vi "Validate ROI arrays.vi"(7 "[ROI vis]":refnum<vi>, 9 "Old Value":T1 caption="Old value" {"ROI number" min=1 format="ROI %.0f"}, 11 "New Value":T1 caption="New value" {"ROI number" min=1 format="ROI %.0f"}) -> (0 "error out":errorcluster, 3 "[ROI #] out":T1 caption="Selected POI" {"ROI number" min=1 format="ROI %.0f"})   [LabVIEW 2013]
uses:
  Typedefs/ROI selector array-ROI vis.ctl
  xcontrol/Interface VIs/Interface typedefs/Interface-ROI selection cluster.ctl
  Typedefs/ROI ID Enum.ctl
  Typedefs/Get-Set-Clear Control.ctl
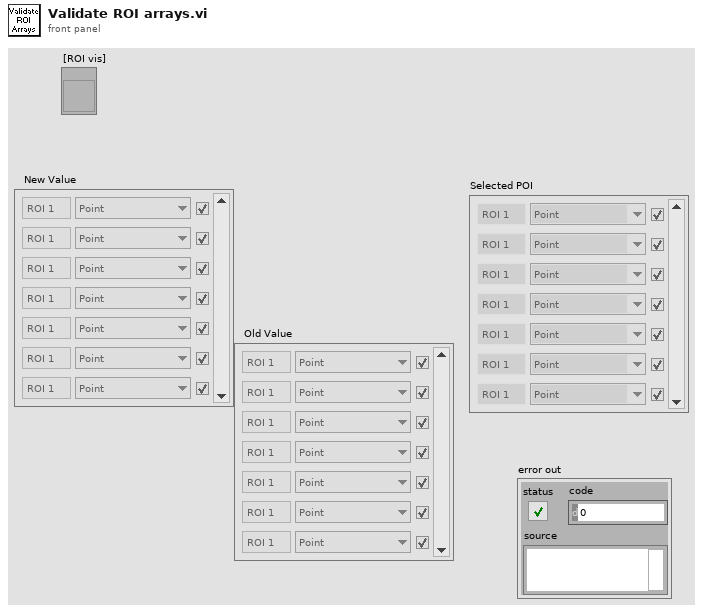
[diagram p1: front panel]
types:
  T1 = typedef "ROI selector array-ROI vis.ctl" = T2[]
  T2 = typedef "Interface-ROI selection cluster.ctl" = cluster{"ROI number":i32, "ROI ID":T3, "Visibility":bool}
  T3 = typedef "ROI ID Enum.ctl" = enum16{"Point", "MiniScan", "Comp. MiniScan", "Rectangle", "Comp. volume", "Arb. plane point"}
  T4 = cluster{"ROI number":i32, "ROI ID":T3, "Visibility":bool}
  T5 = cluster{"ROI number":i32, "ROI ID":T3, "Visibility":bool}[]
  T6 = cluster{"ROI index changed":bool, "ROI ID":bool, "Visibility changed":bool}
  T7 = typedef "Get-Set-Clear Control.ctl" = enum16{"Get", "Set", "Clear"}
  T8 = cluster{"ROI number":bool, "ROI ID":bool, "Visibility":bool}[]
  T9 = typedef "ROI indexes by type.ctl" = cluster{"Indexes of POI":i32[], "Indexes of Miniscans":i32[], "Indexes of? (Provisional)":i32[]}
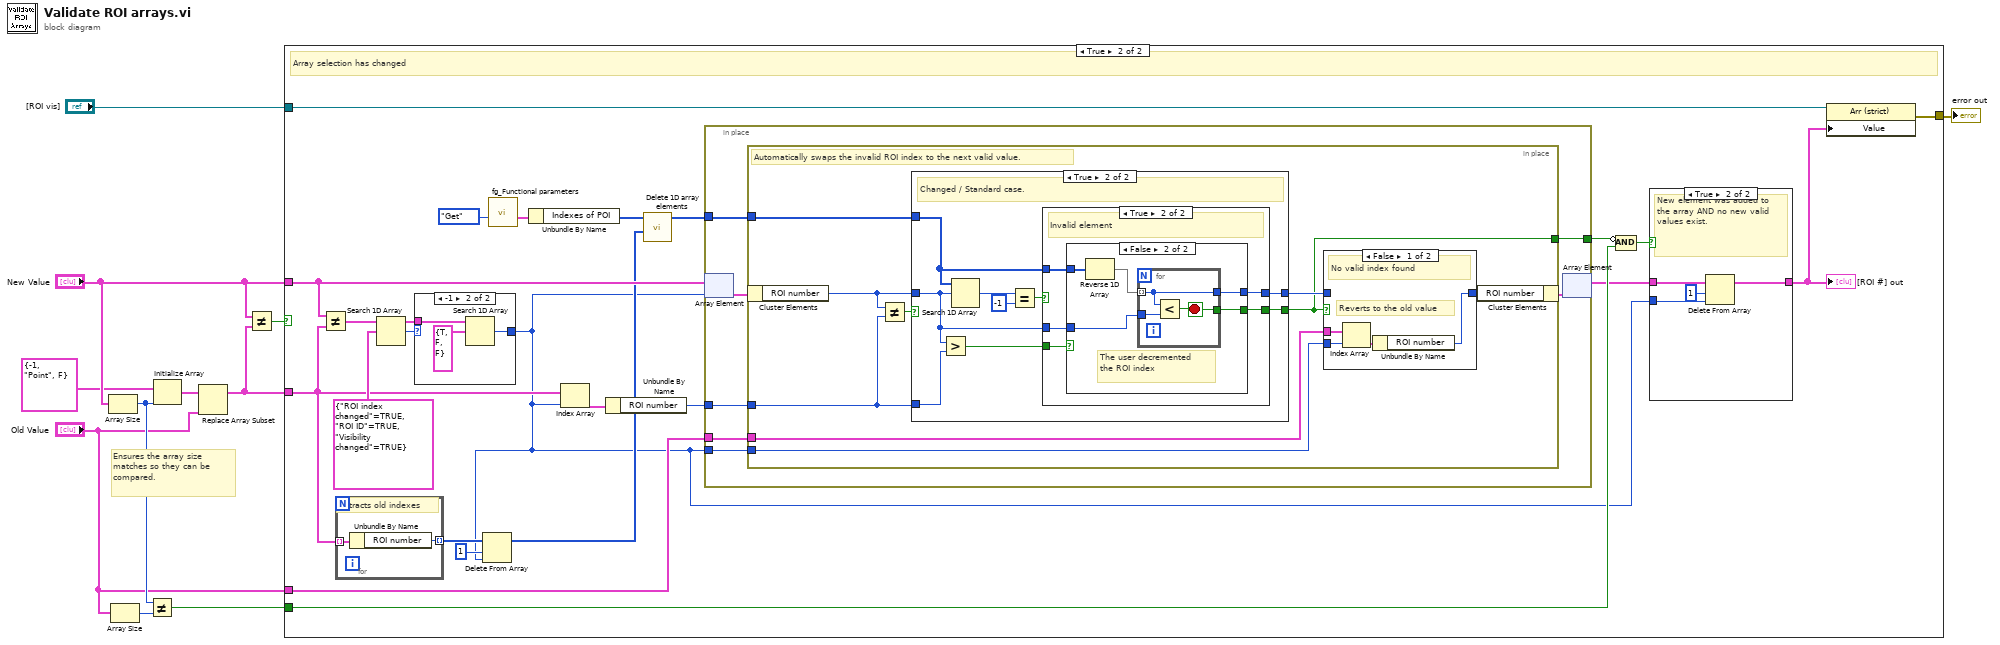
[diagram p0: block diagram]
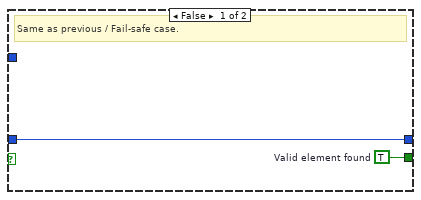
[diagram p5: hidden frame]
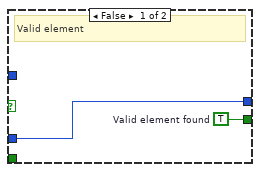
[diagram p6: hidden frame]
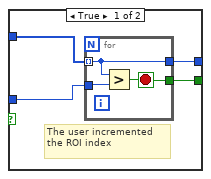
[diagram p7: hidden frame]
diagram:
  # "Ensures the array size matches so they can be compared."
  n1 = Array Size(array="New Value") -> (size(s)=w7:i32)
  n2 = Array Size(array="Old Value") -> (size(s)=w6:i32)
  n3 = Not Equal?(x=w7, y=w6) -> (x != y?=w5:bool)
  n4 = Initialize Array(T4 {"ROI number"=-1, "ROI ID"=enum."Point", "Visibility"=FALSE} ("System Cluster"), w7) -> (w10:T5)
  n5 = Replace Array Subset(array=w10, new element="Old Value") -> (w9:T5)  [unwired: 1 in]
  n6 = Not Equal?(x="New Value", y=w9) -> (x != y?=w11:bool)
  n7 = case shown="True" w11 {
    tunnel: "[ROI vis]" -> [_ w32]
    tunnel: "New Value" -> [_ w26]
    tunnel: w9 -> [_ w25]
    tunnel: w5 -> [_ w19]
    tunnel: "Old Value" -> [_ w14]
    tunnel: [_ w13] -> w3
    frame False {
      # "No change"
    }
    frame True {
      # "Array selection has changed"
      n8 = Not Equal?(x=w26, y=w25) -> (x != y?=w29:T8)
      n9 = for {
        tunnel: w25 -> [w41] mode=indexing
        tunnel: [w40] -> w24 mode=indexing
        # "Extracts old indexes"
        n10 = Unbundle By Name(w41) -> ("ROI number"=w40:i32)
      }
      n11 = Search 1D Array(1D array=w29, element=T6 {"ROI index changed"=TRUE, "ROI ID"=TRUE, "Visibility changed"=TRUE} ("POI sel & vis")) -> (index of element=w30:i32)  [unwired: 1 in]
      n12 = case shown="-1" w30 {
        selector: w30 -> [w96 _]
        tunnel: w29 -> [_ w99]
        tunnel: [w96 w98] -> w12
        frame Default {
        }
        frame -1 {
          n13 = Search 1D Array(1D array=w99, element=T6 {"ROI index changed"=TRUE, "ROI ID"=FALSE, "Visibility changed"=FALSE} ("POI sel & vis")) -> (index of element=w98:i32)  [unwired: 1 in]
        }
      }
      n14 = Delete From Array "Delete From Array"(array=w24, length=1, index=w12) -> (array with subset deleted=w22:i32[])  [unwired: 1 out]
      n15 = call "fg_Functional parameters.vi"("Function"=Get-Set-Clear_Control."Get") -> ("ROI indexes by type"=w33:T9)  [unwired: 7 in, 3 out]
      n16 = Unbundle By Name(w33) -> ("Indexes of POI"=w20:i32[])
      n17 = Index Array(array=w25, index=w12) -> (element=w28:T4)
      n18 = Unbundle By Name(w28) -> ("ROI number"=w27:i32)
      n19 = call "Delete 1D array elements.vi"("Elements to delete"=w22, "Input array"=w20) -> ("Array w elements deleted"=w21:i32[])  [unwired: 9 in]
      n20 = in-place {
        in-place-border: w21 -> [w48]
        in-place-border: w27 -> [w45]
        in-place-border: w14 -> [w44]
        in-place-border: w12 -> [w43]
        in-place-border: [w42] -> w18
        n21 = in-place-array #1(w26, w12) -> (w47:T2)
        n22 = in-place {
          in-place-border: w48 -> [w54]
          in-place-border: w45 -> [w55]
          in-place-border: w44 -> [w53]
          in-place-border: w43 -> [w52]
          in-place-border: [w49] -> w42
          # "Automatically swaps the invalid ROI index to the next valid value."
          n23 = in-place-cluster #2(w47) -> ("ROI number"=w57:i32)
          n24 = Not Equal?(x=w57, y=w55) -> (x != y?=w56:bool)
          n25 = case shown="True" w56 {
            tunnel: [w64 w70] -> w51
            tunnel: w54 -> [_ w69]
            tunnel: w57 -> [w64 w68]
            tunnel: w55 -> [_ w67]
            tunnel: [w63 w65] -> w49
            frame False {
              w63 = TRUE  # Valid element found
              # "Same as previous / Fail-safe case."
            }
            frame True {
              # "Changed / Standard case."
              n26 = Greater?(x=w68, y=w67) -> (0:w66:bool)
              n27 = Search 1D Array(1D array=w69, element=w68) -> (index of element=w73:i32)  [unwired: 1 in]
              n28 = Equal?(x=w73, y=-1) -> (x = y?=w71:bool)
              n29 = case shown="True" w71 {
                tunnel: [w75 w78] -> w70
                tunnel: w68 -> [w75 w79]
                tunnel: w69 -> [_ w80]
                tunnel: w66 -> [_ w77]
                tunnel: [w74 w76] -> w65
                frame False {
                  w74 = TRUE  # Valid element found
                  # "Valid element"
                }
                frame True {
                  # "Invalid element"
                  n30 = case shown="False" w77 {
                    tunnel: w80 -> [w84 w92]
                    tunnel: w79 -> [w83 w91]
                    tunnel: [w82 w90] -> w78
                    tunnel: [w81 w88] -> w76
                    frame True {
                      # "The user incremented the ROI index"
                      n31 = for {
                        tunnel: w84 -> [w86] mode=indexing
                        tunnel: w83 -> [w87]
                        tunnel: [w86] -> w82
                        tunnel: [w85] -> w81
                        stop <- w85 stop-if-true
                        n32 = Greater?(x=w86, y=w87) -> (0:w85:bool)
                      }
                    }
                    frame False {
                      # "The user decremented the ROI index"
                      n33 = Reverse 1D Array(array=w92) -> (reversed array=w89:i32[])
                      n34 = for {
                        tunnel: w89 -> [w94] mode=indexing
                        tunnel: w91 -> [w95]
                        tunnel: [w94] -> w90
                        tunnel: [w93] -> w88
                        stop <- w93 stop-if-true
                        n35 = Less?(x=w94, y=w95) -> (x < y?=w93:bool)
                      }
                    }
                  }
                }
              }
            }
          }
          n36 = case shown="False" w49 {
            tunnel: w53 -> [w61 _]
            tunnel: w52 -> [w60 _]
            tunnel: w51 -> [_ w62]
            tunnel: [w58 w62] -> w50
            frame False {
              # "Reverts to the old value"
              # "No valid index found"
              n37 = Index Array(array=w61, index=w60) -> (element=w59:T2)
              n38 = Unbundle By Name(w59) -> ("ROI number"=w58:i32)
            }
            frame True {
              # "Valid index found"
            }
          }
          n39 = in-place-cluster #2("ROI number"=w50) -> (w46:T2)
        }
        n40 = in-place-array #1(w46) -> (w16:T1)  [unwired: 1 out]
      }
      n41 = Compound Arithmetic op=AND(invert w18, w19) -> (w17:bool)
      n42 = case shown="True" w17 {
        tunnel: w16 -> [w35 w39]
        tunnel: [w35 w38] -> w15
        tunnel: w12 -> [_ w37]
        frame False {
          # "Number of array elements did not change, or valid elements exist."
        }
        frame True {
          # "New element was added to the array AND no new valid values exist."
          n43 = Delete From Array(array=w39, length=1, index=w37) -> (array with subset deleted=w38:T1)  [unwired: 1 out]
        }
      }
      "[ROI #] out" <- w15
      n44 = property class="Arr (strict)"(reference=w32, "Value"=w15) -> (error out=w13:errorcluster)  [unwired: 1 in, 1 out]
    }
  }
  "error out" <- w3
